vi "Simple Test.vi"() -> ()   [LabVIEW 2016, in "xy_utilities.lvlib"]
uses:
  xy_utilities.lvlib
  Derivative (single).vi
  Multiply float (single).vi
  Subset (single).vi
  Sort (single).vi
panel:
  out "Homegrown \"Slope\" Differential XY Data":cluster{"X-array":dbl[], "Y-array":dbl[]}[](graph)
  in  "period (V)":dbl[](array[numeric]) format="%#_6p"
  in  "max":dbl format="%#_6p"
  in  "min":dbl format="%#_6p"
  out "Homegrown \"Slope\" Differential":dbl[][](graph)
  out "Zero Phase Filter  + 2nd Order Central Differential":dbl[][](graph)
  out "Zero Phase Filter + 2nd Order Central Differential XY Data":cluster{"X-array":dbl[], "Y-array":dbl[]}[](graph)
  out "Filtered XY Data (example)":cluster{"X-array":dbl[], "Y-array":dbl[]}[](graph)
  out "XY Data":cluster{"X-array":dbl[], "Y-array":dbl[]}(graph)
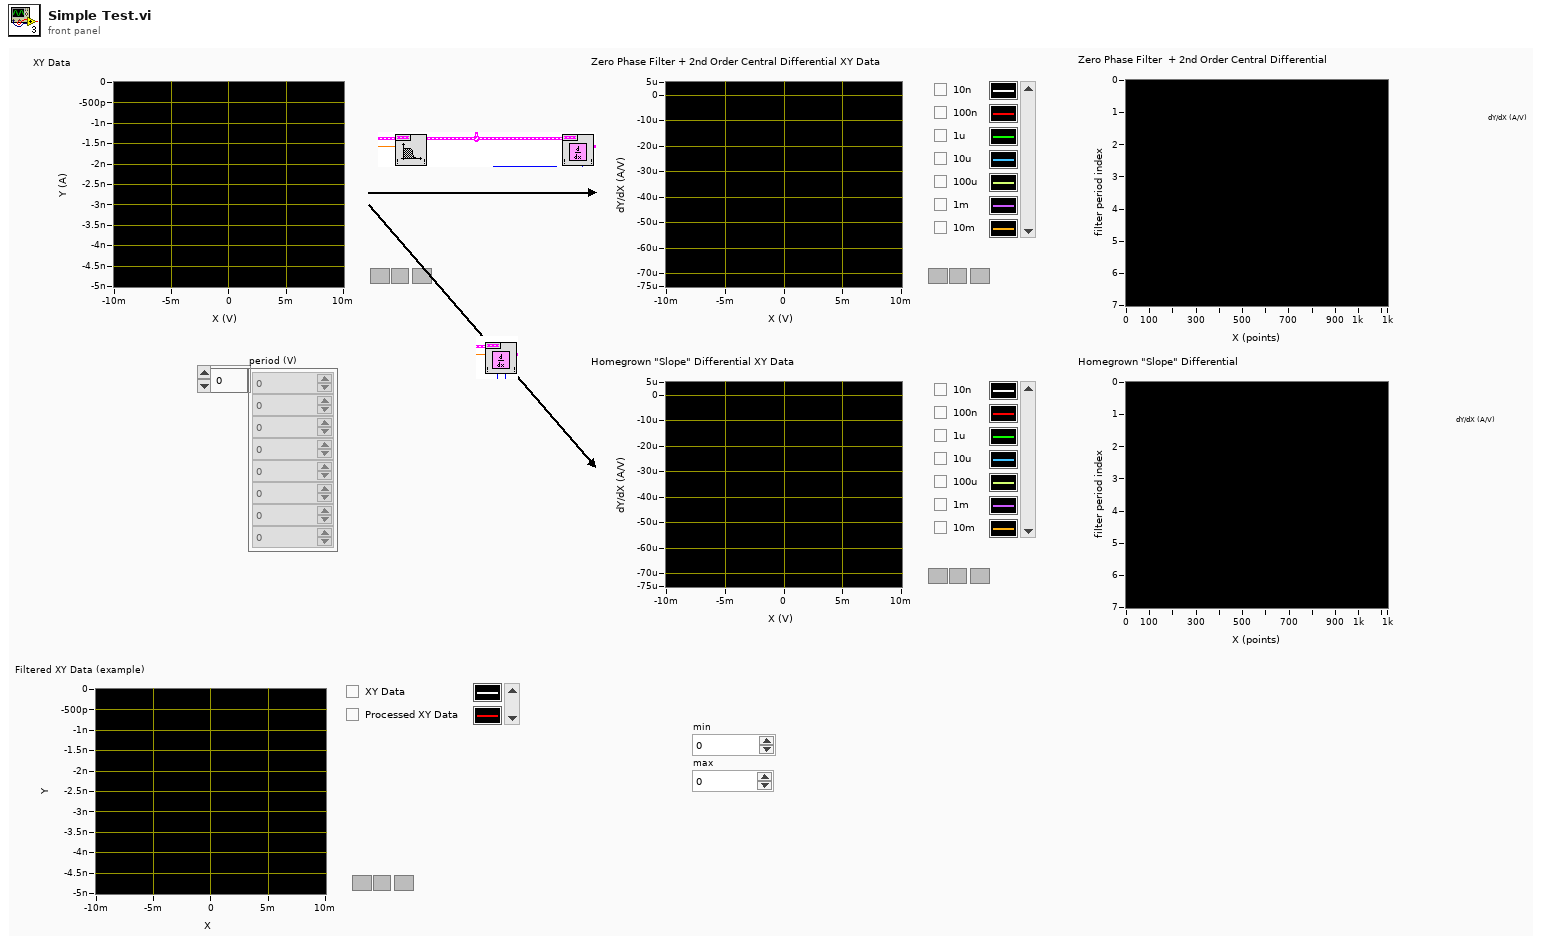
[diagram p1: front panel]
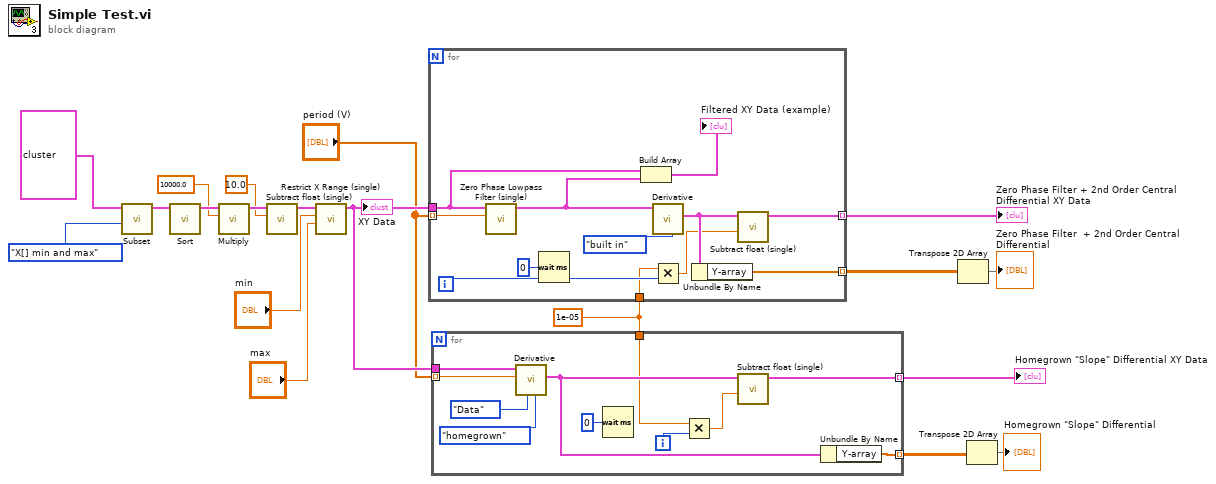
[diagram p0: block diagram]
diagram:
  w1 = 1e-05 ("x")
  n1 = call-poly "Subset.vi"("Subset Method"=enum16{"Slider (%)", "X[] min and max"}."X[] min and max", "XY-data"=cluster{"X Array":dbl[], "Y Array":dbl[]} {"X Array"=array[2480 elements], "Y Array"=array[2480 elements]} ("XY-data horizontal")) -> ("XY-data out"=w12:cluster{"X-array":dbl[], "Y-array":dbl[]})  [unwired: 8 in, 1 out]
  n2 = call-poly "Sort.vi"("XY-data"=w12) -> ("Sorted XY-data out"=w11:cluster{"X-array":dbl[], "Y-array":dbl[]})  [unwired: 9 in, 1 out]
  n3 = call-poly "Multiply.vi"("x (1)"=10000.0 ("x"), "XY-data"=w11) -> ("XY-data out"=w10:cluster{"X-array":dbl[], "Y-array":dbl[]})  [unwired: 8 in, 1 out]
  n4 = call "Subtract float (single).vi"("x (0)"=10.0 ("x"), "XY-data"=w10) -> ("XY-data out"=w9:cluster{"X-array":dbl[], "Y-array":dbl[]})  [unwired: 8 in, 1 out]
  n5 = call "Restrict X Range (single).vi"("X Max"="max", "X Min"="min", "XY-data"=w9) -> ("XY-data out"=w5:cluster{"X-array":dbl[], "Y-array":dbl[]})  [unwired: 7 in, 1 out]
  "XY Data" <- w5
  n6 = for {
    tunnel: "period (V)" -> [w25] mode=indexing
    tunnel: w5 -> [w30]
    tunnel: [w23] -> w19 mode=indexing
    tunnel: [w27] -> w4 mode=indexing
    tunnel: w1 -> [w20]
    i -> [w24]
    n7 = call "Zero Phase Lowpass Filter (single).vi"("cutoff period"=w25, "XY-data"=w30) -> ("XY-data out"=w28:cluster{"X-array":dbl[], "Y-array":dbl[]})  [unwired: 8 in, 1 out]
    n8 = Wait (ms)(milliseconds to wait=u32 0) -> ()  [unwired: 1 out]
    n9 = Build Array(w30, w28) -> (→"Filtered XY Data (example)":cluster{"X-array":dbl[], "Y-array":dbl[]}[])
    n10 = call-poly "Derivative.vi"(4:enum16{"built in", "homegrown"}."built in" ("Subset Method"), "XY-data"=w28) -> ("Differential out"=w22:cluster{"X-array":dbl[], "Y-array":dbl[]})  [unwired: 7 in, 2 out]
    n11 = Multiply(x=w20, y=w24) -> (x*y=w21:dbl)
    n12 = Unbundle By Name(w22) -> ("Y-array"=w27:dbl[])
    n13 = call "Subtract float (single).vi"("y (0)"=w21, "XY-data"=w22) -> ("XY-data out"=w23:cluster{"X-array":dbl[], "Y-array":dbl[]})  [unwired: 8 in, 1 out]
  }
  "Zero Phase Filter + 2nd Order Central Differential XY Data" <- w19
  n14 = for {
    tunnel: w5 -> [w40]
    tunnel: [w42] -> w16 mode=indexing
    tunnel: "period (V)" -> [w38] mode=indexing
    tunnel: [w33] -> w2 mode=indexing
    tunnel: w1 -> [w32]
    i -> [w35]
    n15 = call-poly "Derivative.vi"(4:enum16{"built in", "homegrown"}."homegrown" ("Subset Method"), "Interval Units"=enum16{"Points", "Data"}."Data", "Interval (h)"=w38, "XY-data"=w40) -> ("Differential out"=w36:cluster{"X-array":dbl[], "Y-array":dbl[]})  [unwired: 5 in, 2 out]
    n16 = Wait (ms)(milliseconds to wait=u32 0) -> ()  [unwired: 1 out]
    n17 = Multiply(x=w32, y=w35) -> (x*y=w34:dbl)
    n18 = call "Subtract float (single).vi"("y (0)"=w34, "XY-data"=w36) -> ("XY-data out"=w33:cluster{"X-array":dbl[], "Y-array":dbl[]})  [unwired: 8 in, 1 out]
    n19 = Unbundle By Name(w36) -> ("Y-array"=w42:dbl[])
  }
  "Homegrown \"Slope\" Differential XY Data" <- w2
  n20 = Transpose 2D Array(2D array=w4) -> (transposed array=→"Zero Phase Filter  + 2nd Order Central Differential":dbl[][])
  n21 = Transpose 2D Array(2D array=w16) -> (transposed array=→"Homegrown \"Slope\" Differential":dbl[][])
